vi "1_0_Function Generator.vi"(0 "Ramp end":dbl=1.0 format="%0.2f", 1 "Ramp start":dbl format="%0.2f", 3 "Chirp Freq 1":dbl format="%0.2f", 4 "Chirp Freq 2":dbl=0.5 format="%0.2f", 5 "Arbitrary Wave Table":dbl[](array[numeric])=[1.0, 2.0, 3.0, 4.0, 5.0, 6.0, 7.0, 0.0] format="%0.2f", 7 "Pulse width":i32=11, 8 "delta t (Sinc pattern)":dbl=0.10000000000000009 format="%0.2f", 9 "duty cycle (%)\n(Square wave)":dbl(knob)=50.0 scale=0.0..100.0, 11 "Samples":i32=128, 12 "Pattern":T1(ring)=enum."Sine wave", 14 "Phase in":dbl(knob) scale=-180.0..180.0, 15 "Frequency":dbl(knob)=200.0 scale=0.0..1000.0 scale format="%#_6p", 16 "Amplitude":dbl(knob)=1.0 scale=0.0..10.0, 17 "Delay":i32(knob)=9 scale=0.0..120.0, 20 "reset phase":bool=TRUE, 21 "standard deviation\n(Gaussian white noise)":dbl=1.0000000000000002 format="%0.2f", 23 "spectral amplitude\n(Periodic Random Noise)":dbl=1.0 format="%0.2f", 24 "order\n(Gamma Noise)":i32=1, 25 "mean\n(Poisson Noise)":dbl=1.0 format="%0.2f", 26 "trial probability\n(Binomial Noise)":dbl=0.5 format="%.2f", 27 "trials (Binomial Noise)":i32=5) -> (13 "?":dbl[](graph)=[0.0, 0.12533323356430426, 0.2486898871648548, 0.368124552684678, 0.48175367410171527, 0.5877852522924731, 0.6845471059286887, 0.7705132427757893, 0.8443279255020152, 0.9048270524660196, 0.9510565162951536, 0.9822872507286887, 0.9980267284282716, 0.9980267284282716, 0.9822872507286886, 0.9510565162951534, 0.9048270524660194, 0.8443279255020147, 0.770513242775789, 0.6845471059286885, 0.5877852522924731, 0.4817536741017155, 0.36812455268467836, 0.2486898871648554, 0.1253332335643051, 1.045116684167402e-15, -0.125333233564303, -0.24868988716485338, -0.3681245526846764, -0.48175367410171366, -0.5877852522924715, -0.6845471059286871, -0.7705132427757877, -0.8443279255020136, -0.9048270524660184, -0.9510565162951526, -0.982287250728688, -0.9980267284282713, -0.9980267284282718, -0.9822872507286894, -0.9510565162951549, -0.9048270524660214, -0.8443279255020175, -0.7705132427757923, -0.6845471059286922, -0.5877852522924772, -0.4817536741017199, -0.368124552684683, -0.24868988716486026, -0.12533323356431006, -6.0588470005007444e-15, 0.12533323356429804, 0.24868988716484852, 0.36812455268467176, 0.4817536741017093, 0.5877852522924674, 0.6845471059286834, 0.7705132427757845, 0.844327925502011, 0.9048270524660161, 0.9510565162951511, 0.9822872507286872, 0.998026728428271, 0.9980267284282721, 0.9822872507286904, 0.9510565162951564, 0.9048270524660235, 0.8443279255020202, 0.7705132427757954, 0.6845471059286958, 0.5877852522924812, 0.48175367410172426, 0.3681245526846877, 0.24868988716486418, 0.12533323356431306, 8.096442353361377e-15, -0.125333233564297, -0.24868988716484847, -0.36812455268467265, -0.48175367410171094, -0.5877852522924698, -0.6845471059286863, -0.7705132427757876, -0.8443279255020142, -0.9048270524660191, -0.9510565162951535, -0.9822872507286888, -0.9980267284282717, -0.9980267284282714, -0.9822872507286882, -0.9510565162951524, -0.9048270524660176, -0.8443279255020122, -0.7705132427757853, -0.6845471059286836, -0.5877852522924669, -0.48175367410170783, -0.3681245526846693, -0.248689887164845, -0.12533323356429343, 1.1693120430256165e-14, 0.12533323356431664, 0.24868988716486765, 0.368124552684691, 0.4817536741017283, 0.5877852522924858, 0.6845471059287006, 0.7705132427758002, 0.8443279255020247, 0.9048270524660276, 0.9510565162951596, 0.9822872507286925, 0.9980267284282729, 0.9980267284282702, 0.9822872507286844, 0.9510565162951463, 0.9048270524660091, 0.8443279255020016, 0.7705132427757727, 0.6845471059286692, 0.5877852522924508, 0.48175367410169045, 0.3681245526846509, 0.24868988716482582, 0.1253332335642738, -3.148181585213572e-14, -0.12533323356433626, -0.24868988716488682])   [LabVIEW 2009]
doc: "This program can be can be used to visualize basic signals."
uses:
  Instance          17 30Saved   1_0_Function Generator .vi
  <vilib>/Analysis/NI_AALBase.lvlib
panel:
  out "?":string="Doubling a signal quadruples the Energy. But time shifting a signal has no effect on the signal."
  out "ENERGY":dbl=62.577555079413656 format="%#_4g"
  out "POWER":dbl=0.4888871490579192 format="%#_4g"
  in  "Time Delay (seconds)":dbl(slide) scale=0.0..1.0
  in  "Sampling freq.":dbl=10000.0 format="%#_6p"
  in  "stop":bool
  # "Program Developed by Indranil Sinharoy"
  # "Function Generator"
  # "Arbitrary Wave Pattern"
  # "Pulse"
  # "Sinc Pattern"
  # "Square Wave"
  # "Ramp"
  # "Chirp Pattern"
  # "Gaussian White Noise"
  # "Periodic Random Noise"
  # "Gamma Noise"
  # "Poisson Noise"
  # "Binomial Noise"
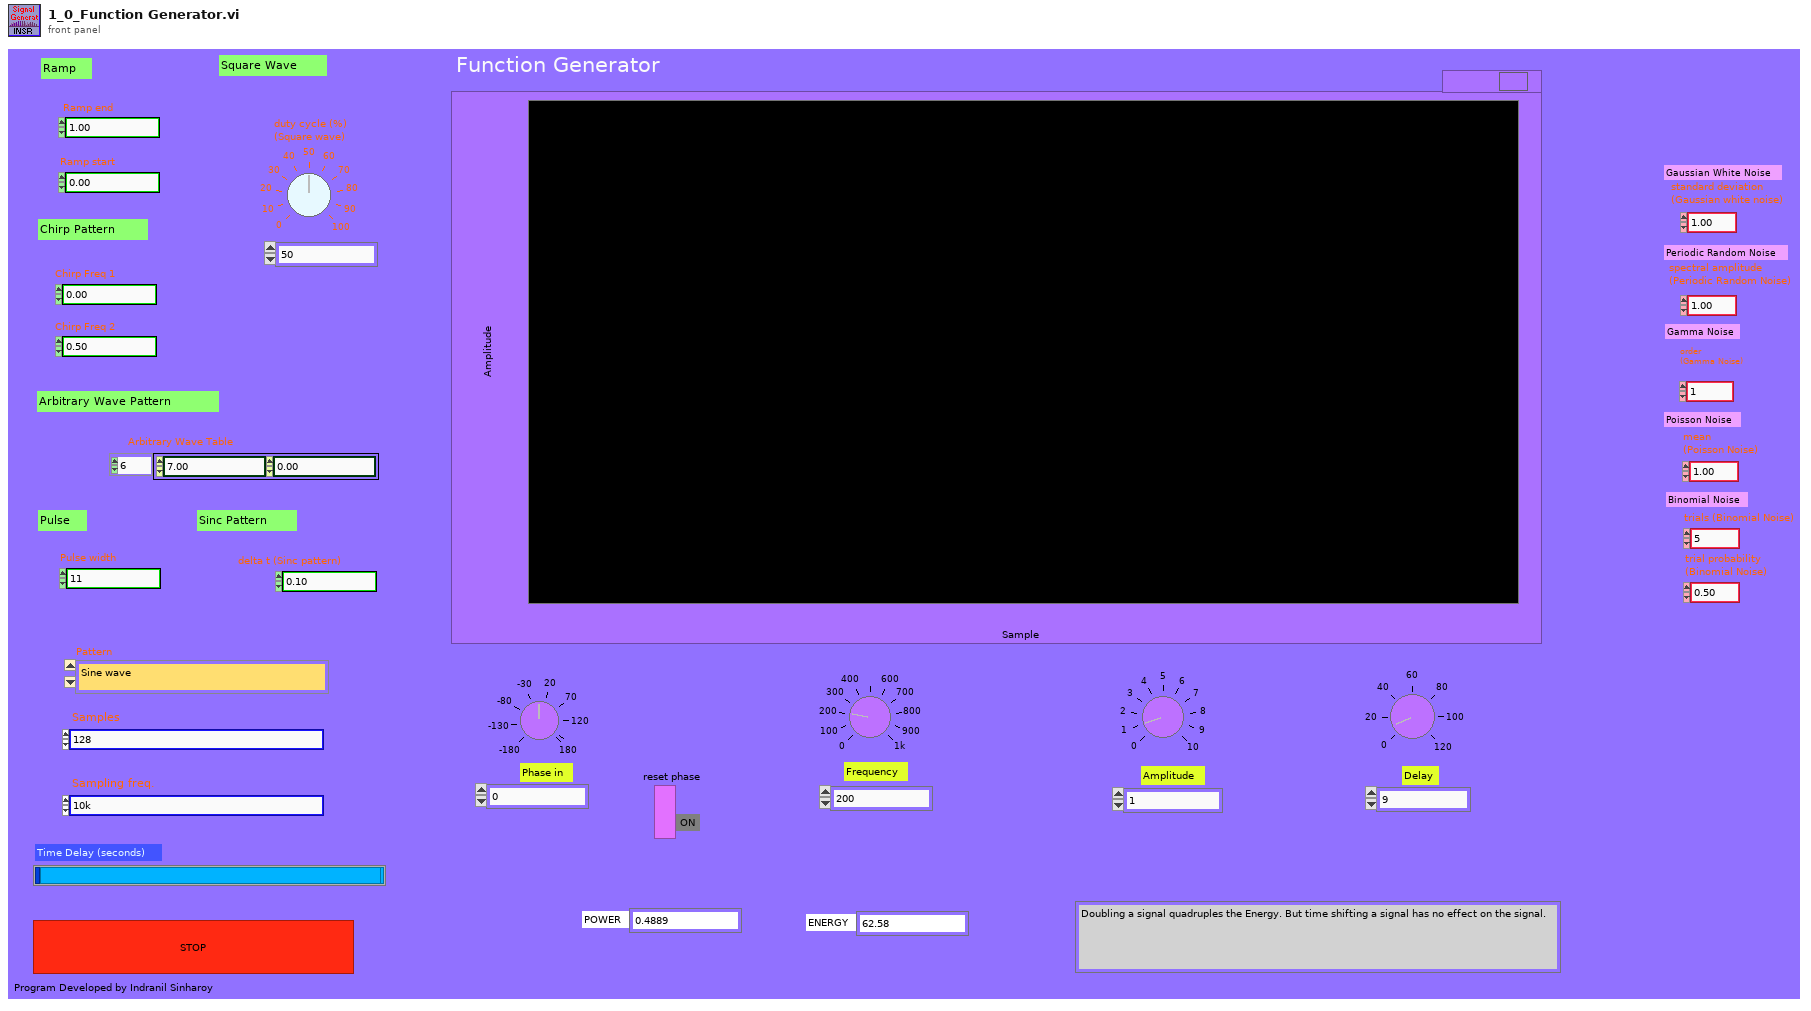
[diagram p1: front panel]
types:
  T1 = enum16{"Impulse", "Ramp", "Pulse", "Chirp Pattern", "Sinc Pattern", "Sine wave", "Square wave", "Triangle wave", "Sawtooth wave", "Arbitrary wave", "Uniform White Noise", "Gaussian White Noise", "Periodic Random Noise", "Gamma Noise", "Poisson Noise", "Binomial Noise"}
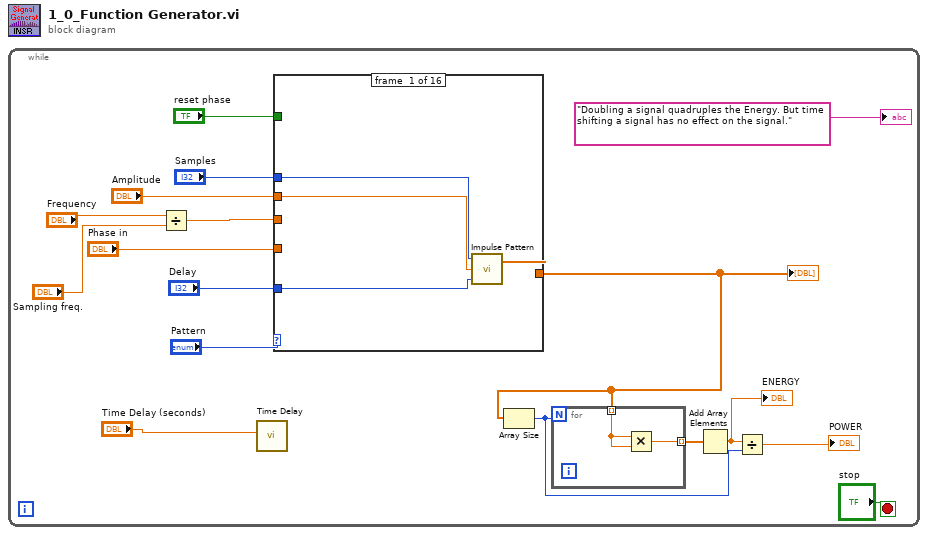
[diagram p0: block diagram]
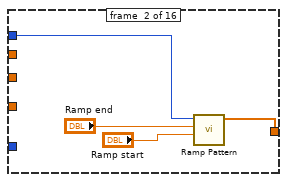
[diagram p2: hidden frame]
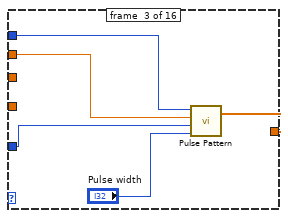
[diagram p3: hidden frame]
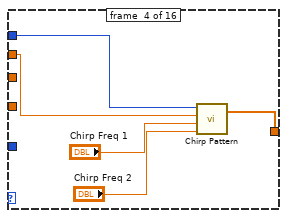
[diagram p4: hidden frame]
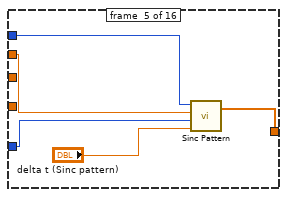
[diagram p5: hidden frame]
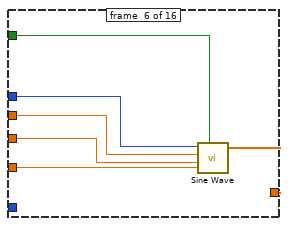
[diagram p6: hidden frame]
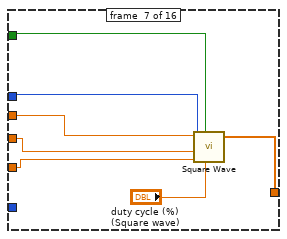
[diagram p7: hidden frame]
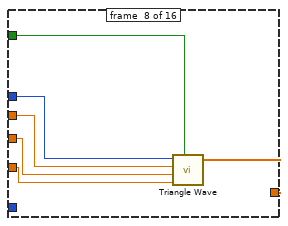
[diagram p8: hidden frame]
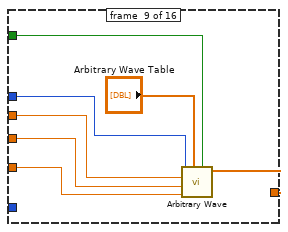
[diagram p9: hidden frame]
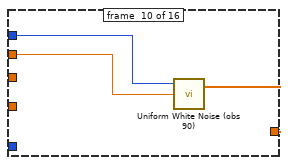
[diagram p10: hidden frame]
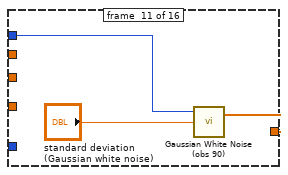
[diagram p11: hidden frame]
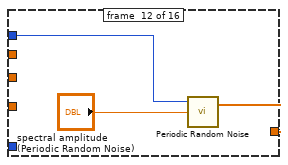
[diagram p12: hidden frame]
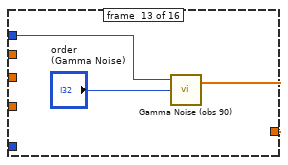
[diagram p13: hidden frame]
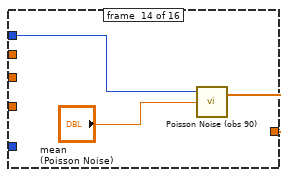
[diagram p14: hidden frame]
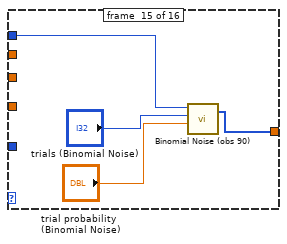
[diagram p15: hidden frame]
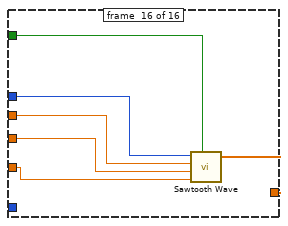
[diagram p16: hidden frame]
diagram:
  n1 = while {
    stop <- "stop" stop-if-true
    n2 = Divide(x="Frequency", y="Sampling freq.") -> (x/y=w9:dbl)
    n3 = call "Time Delay"("Delay Time (s)"="Time Delay (seconds)") -> ()  [unwired: 10 in, 1 out]
    n4 = case shown="\"Arbitrary wave\"" "Pattern" {
      tunnel: "Samples" -> [w23 w27 w31 w36 w42 w48 w53 w56 w67 w70 w73 w76 w79 w82 w86 w92]
      tunnel: "Amplitude" -> [w22 _ w30 w35 w41 w47 w52 w57 w66 w69 _ _ _ _ _ w91]
      tunnel: [w21 w26 w32 w37 w38 w46 w55 w61 w63 w71 w74 w77 w80 w83 w87 w88] -> w6
      tunnel: "Delay" -> [w20 _ w29 _ w40 _ _ _ _ _ _ _ _ _ _ _]
      tunnel: w9 -> [_ _ _ _ _ w45 w51 w58 w65 _ _ _ _ _ _ w90]
      tunnel: "Phase in" -> [_ _ _ _ _ w44 w50 w59 w64 _ _ _ _ _ _ w89]
      tunnel: "reset phase" -> [_ _ _ _ _ w43 w54 w60 w62 _ _ _ _ _ _ w93]
      frame #0 {
        n5 = call <vilib>:"Impulse Pattern.vi"("delay"=w20, "amplitude"=w22, "samples"=w23) -> ("Impulse Pattern"=w21:dbl[])  [unwired: 1 out]
      }
      frame #1 {
        n6 = call <vilib>:"Ramp Pattern.vi"("start"="Ramp start", "end"="Ramp end", "samples"=w27) -> ("Ramp Pattern"=w26:dbl[])  [unwired: 7 in, 1 out]
      }
      frame #2 {
        n7 = call <vilib>:"Pulse Pattern.vi"("width"="Pulse width", "delay"=w29, "amplitude"=w30, "samples"=w31) -> ("Pulse Pattern"=w32:dbl[])  [unwired: 1 out]
      }
      frame #3 {
        n8 = call <vilib>:"Chirp Pattern.vi"("f2"="Chirp Freq 2", "f1"="Chirp Freq 1", "amplitude"=w35, "samples"=w36) -> ("Chirp Pattern"=w37:dbl[])  [unwired: 1 out]
      }
      frame #4 {
        n9 = call <vilib>:"Sinc Pattern.vi"("delta t"="delta t (Sinc pattern)", "delay"=w40, "amplitude"=w41, "samples"=w42) -> ("Sinc Pattern"=w38:dbl[])  [unwired: 1 out]
      }
      frame #5 {
        n10 = call <vilib>:"Sine Wave.vi"("samples"=w48, "amplitude"=w47, "frequency"=w45, "phase in"=w44, "reset phase"=w43) -> ("sine wave"=w46:dbl[])  [unwired: 2 out]
      }
      frame #6 {
        n11 = call <vilib>:"Square Wave.vi"("samples"=w53, "reset phase"=w54, "amplitude"=w52, "frequency"=w51, "duty cycle (%)"="duty cycle (%)\n(Square wave)", "phase in"=w50) -> ("square wave"=w55:dbl[])  [unwired: 2 out]
      }
      frame #7 {
        n12 = call <vilib>:"Triangle Wave.vi"("samples"=w56, "amplitude"=w57, "frequency"=w58, "phase in"=w59, "reset phase"=w60) -> ("triangle wave"=w61:dbl[])  [unwired: 2 out]
      }
      frame #8 {
        n13 = call <vilib>:"Arbitrary Wave.vi"("reset phase"=w62, "Wave Table"="Arbitrary Wave Table", "phase in"=w64, "frequency"=w65, "amplitude"=w66, "samples"=w67) -> ("arbitrary wave"=w63:dbl[])  [unwired: 1 in, 2 out]
      }
      frame #9 {
        n14 = call <vilib>:"Uniform White Noise (obs 90).vi"("amplitude"=w69, "samples"=w70) -> ("uniform white noise"=w71:dbl[])  [unwired: 1 in, 1 out]
      }
      frame #10 {
        n15 = call <vilib>:"Gaussian White Noise (obs 90).vi"("standard deviation"="standard deviation\n(Gaussian white noise)", "samples"=w73) -> ("Gaussian noise pattern"=w74:dbl[])  [unwired: 1 in, 1 out]
      }
      frame #11 {
        n16 = call <vilib>:"Periodic Random Noise.vi"("spectral amplitude"="spectral amplitude\n(Periodic Random Noise)", "samples"=w76) -> ("periodic random noise"=w77:dbl[])  [unwired: 1 in, 1 out]
      }
      frame #12 {
        n17 = call <vilib>:"Gamma Noise (obs 90).vi"("order"="order\n(Gamma Noise)", "samples"=w79) -> ("gamma noise"=w80:dbl[])  [unwired: 1 in, 1 out]
      }
      frame #13 {
        n18 = call <vilib>:"Poisson Noise (obs 90).vi"("mean"="mean\n(Poisson Noise)", "samples"=w82) -> ("poisson noise"=w83:dbl[])  [unwired: 1 in, 1 out]
      }
      frame #14 {
        n19 = call <vilib>:"Binomial Noise (obs 90).vi"("trial probability"="trial probability\n(Binomial Noise)", "trials"="trials (Binomial Noise)", "samples"=w86) -> ("binomial noise"=w87:u32[])  [unwired: 1 in, 1 out]
      }
      frame #15 {
        n20 = call <vilib>:"Sawtooth Wave.vi"("samples"=w92, "amplitude"=w91, "frequency"=w90, "phase in"=w89, "reset phase"=w93) -> ("sawtooth wave"=w88:dbl[])  [unwired: 2 out]
      }
    }
    "?" <- w6
    n21 = Array Size(array=w6) -> (size(s)=w3:i32)
    n22 = for {
      N: w3 -> [_]
      tunnel: w6 -> [w19] mode=indexing
      tunnel: [w18] -> w5 mode=indexing
      n23 = Multiply(x=w19, y=w19) -> (x*y=w18:dbl)
    }
    n24 = Add Array Elements(numeric array=w5) -> (sum=w2:dbl)
    "ENERGY" <- w2
    n25 = Divide(x=w2, y=w3) -> (x/y=→"POWER":dbl)
    "?" <- "Doubling a signal quadruples the Energy. But time shifting a signal has no effect on the signal."
  }
